vi "Avery Weight Tronix Driver.vi"(8 "error in (no error)":errorcluster, 11 "Modbus master in":refnum<class "Modbus Master.lvclass">) -> (0 "error out":errorcluster, 1 "Avery Weigth Tronix Data":string[][](array[string]), 2 "Weight Output":T1={"Weight"=29.799999237060547, "Units"="Lbs"}, 3 "Modbus master out":refnum<class "Modbus Master.lvclass">)   [LabVIEW 2016]
uses:
  Type Definitions/Avery Weight Tronix Weight.ctl
  <vilib>/NI/Modbus Library/API/Master/Modbus Master.lvclass
panel:
  in  "Tab Control":enum32{"Page 1", "Page 2"}(tab)
  out "Gross Weight":sgl=29.8
  # "TCP Parameters"
  # "Data to write to the slave"
  # "Slave Read-only Registers"
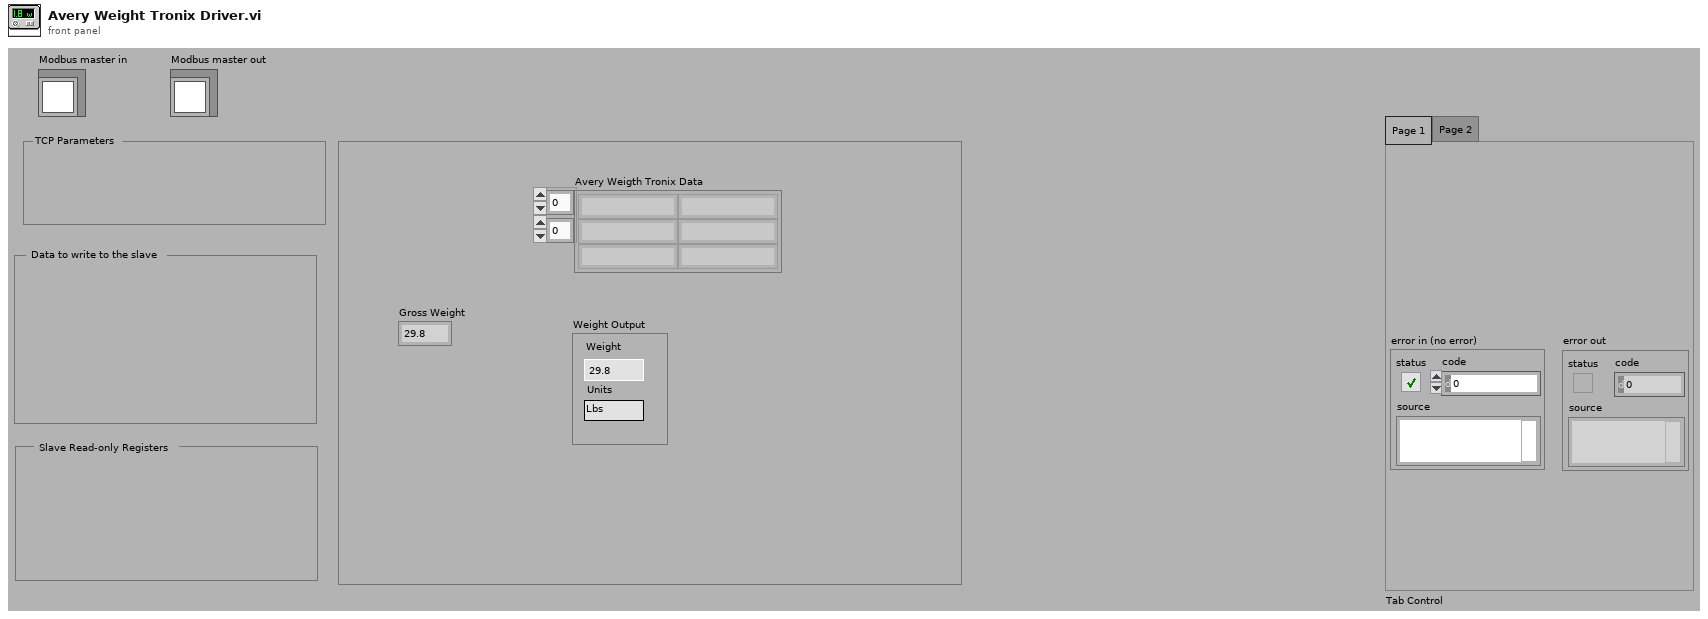
[diagram p1: front panel]
types:
  T1 = typedef "Avery Weight Tronix Weight.ctl" = cluster{"Weight":dbl, "Units":string}
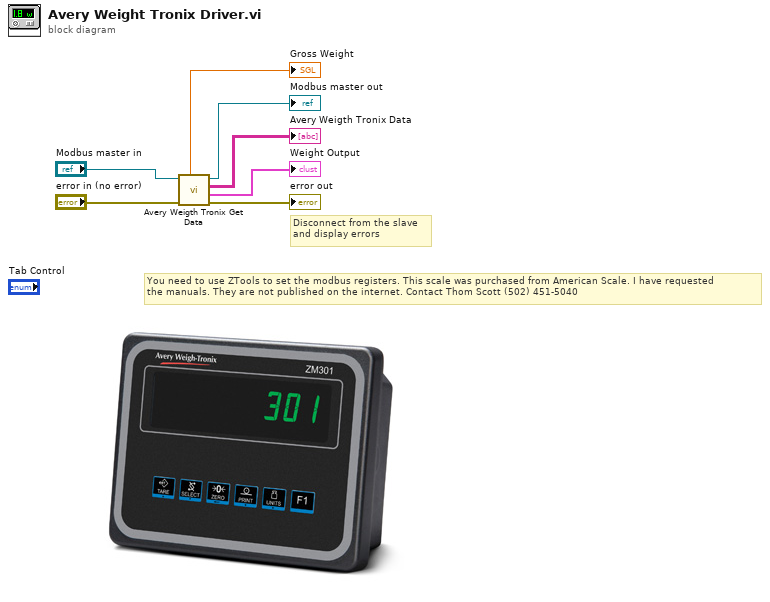
[diagram p0: block diagram]
diagram:
  # "You need to use ZTools to set the modbus registers. This scale was purchased from American Scale. I have requested\nthe manuals. They are not published on the internet. Contact Thom Scott (502) 451-5040"
  # "Disconnect from the slave\nand display errors"
  n1 = call "Avery Weigth Tronix Get Data.vi"("error in (no error)"="error in (no error)", "Modbus master in"="Modbus master in") -> ("error out"=→"error out":errorcluster, "Weight out"=→"Weight Output":T1, "Avery Weigth Tronix Data"=→"Avery Weigth Tronix Data":string[][], "Modbus master out"=→"Modbus master out":refnum<class "Modbus Master.lvclass">, "Gross Weight"=→"Gross Weight":sgl)  [unwired: 5 in]
